vi "__FilterSet_EIDChange.vi"(0 "Param in":cluster{"mode":u8, "AccCode":u32, "AccMask":u32}, 5 "CtrlRef":T1, 7 "IDRef":refnum<vi>[](array[refnum]), 9 "EIDRef":refnum<vi>[](array[refnum]), 11 "error in (no error)":errorcluster, 12 "IDRef 2":refnum<vi>[](array[refnum]), 13 "EIDRef 2":refnum<vi>[](array[refnum])) -> (4 "Param out":cluster{"mode":u8, "AccCode":u32, "AccMask":u32}, 15 "error out":errorcluster)   [LabVIEW 2011]
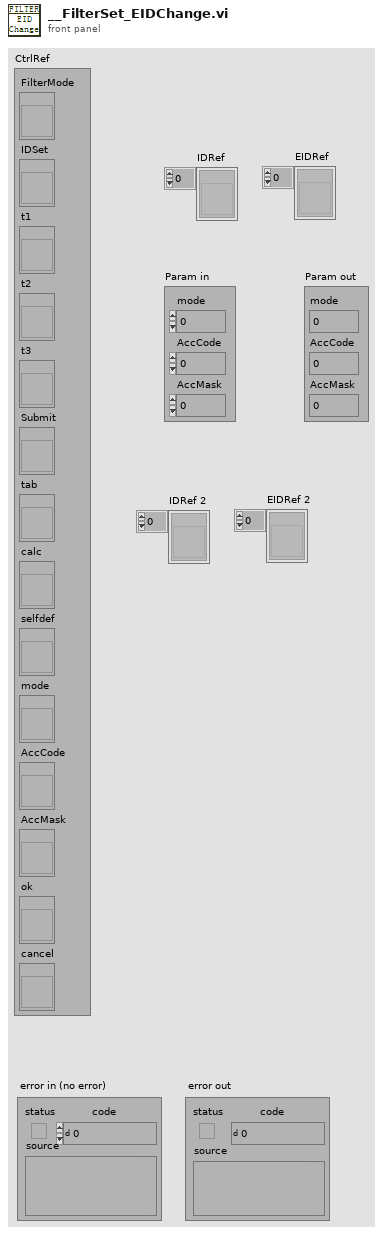
[diagram p1: front panel]
types:
  T1 = cluster{"FilterMode":refnum<vi>, "IDSet":refnum<vi>, "t1":refnum<vi>, "t2":refnum<vi>, "t3":refnum<vi>, "Submit":refnum<vi>, "tab":refnum<vi>, "calc":refnum<vi>, "selfdef":refnum<vi>, "mode":refnum<vi>, "AccCode":refnum<vi>, "AccMask":refnum<vi>, "ok":refnum<vi>, "cancel":refnum<vi>}
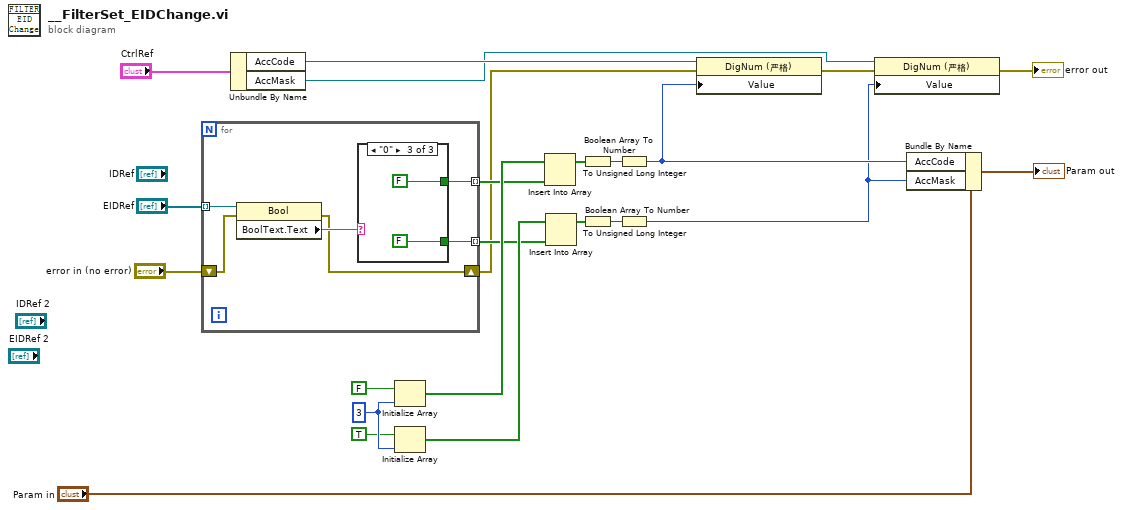
[diagram p0: block diagram]
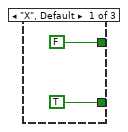
[diagram p2: hidden frame]
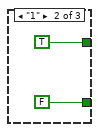
[diagram p3: hidden frame]
diagram:
  w22 = 3 ("维数大小")
  n1 = for {
    tunnel: "EIDRef" -> [w29] mode=indexing
    shift-right: [w24] -> w11
    shift-left: "error in (no error)" -> [w28]
    tunnel: [w26] -> w19 mode=indexing
    tunnel: [w25] -> w17 mode=indexing
    n2 = property class="Bool"(reference=w29, error in=w28) -> (error out=w24:errorcluster, "BoolText.Text"=w27:string)  [unwired: 1 out]
    n3 = case shown="\"0\"" w27 {
      tunnel: [FALSE TRUE FALSE] -> w26
      tunnel: [TRUE FALSE FALSE] -> w25
      frame "X", Default {
      }
      frame "1" {
      }
      frame "0" {
      }
    }
  }
  n4 = Unbundle By Name("CtrlRef") -> ("AccCode"=w12:refnum<vi>, "AccMask"=w9:refnum<vi>)
  n5 = Initialize Array(FALSE, w22) -> (w20:bool[])
  n6 = Initialize Array(TRUE, w22) -> (w18:bool[])
  n7 = Insert Into Array(array=w20, new element=w19) -> (w16:bool[])  [unwired: 1 in]
  n8 = Insert Into Array(array=w18, new element=w17) -> (w15:bool[])  [unwired: 1 in]
  n9 = Boolean Array To Number(Boolean array=w16) -> (number=w14:u32)
  n10 = Boolean Array To Number(Boolean array=w15) -> (number=w13:u32)
  n11 = To Unsigned Long Integer(number=w14) -> (unsigned 32bit integer=w8:u32)
  n12 = To Unsigned Long Integer(number=w13) -> (unsigned 32bit integer=w7:u32)
  n13 = property class="DigNum (严格)"(reference=w12, error in=w11, "Value"=w8) -> (error out=w10:errorcluster)  [unwired: 1 out]
  n14 = property class="DigNum (严格)"(reference=w9, error in=w10, "Value"=w7) -> (error out=→"error out":errorcluster)  [unwired: 1 out]
  n15 = Bundle By Name(cluster="Param in", "AccCode"=w8, "AccMask"=w7) -> (→"Param out":cluster{"mode":u8, "AccCode":u32, "AccMask":u32})
